vi "Send State.vi"(8 "error in (no error)":errorcluster, 11 "LV Server in":refnum<class "LV Server.lvclass">) -> (0 "error out":errorcluster, 3 "LV Server out":refnum<class "LV Server.lvclass">)   [LabVIEW 2020, in "LV Server.lvclass"]
uses:
  LV Server.lvclass
  LV Server.lvclass/LV Server.ctl
  51f6818c-cf3b-408c-aab4-b0425e769b53.vi
  Common/Message ID.ctl
  Common/Common.lvlib
  f25794c6-c553-4325-9ad1-1fe60d8e3a00.vi
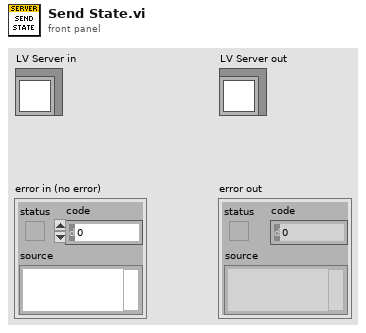
[diagram p1: front panel]
types:
  T1 = typedef "Common.lvlib/Message ID.ctl" = enum16{"Timer State", "Timer Value", "Timer Start", "Timer Pause", "Timer Reset", "Timer Init"}
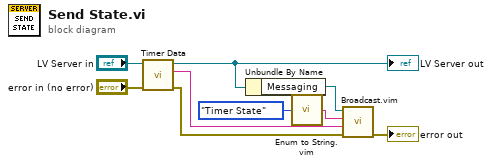
[diagram p0: block diagram]
diagram:
  n1 = call "Timer Data.vi"("error in (no error)"="error in (no error)", "LV Server in"="LV Server in") -> ("error out"=w2:errorcluster, "Timer State"=w5:string, "LV Server out"=w7:refnum<class "LV Server.lvclass">)  [unwired: 6 in, 1 out]
  "LV Server out" <- w7
  n2 = Unbundle By Name(w7) -> ("Messaging"=w6:refnum<class "Manager.lvclass">)
  n3 = call "Enum to String.vim"("Enum"=Message_ID."Timer State" ("Message ID")) -> ("Enum String"=w3:string)
  n4 = call "Broadcast.vim"("error in (no error)"=w2, "Data"=w5, "ID"=w3, "Manager in"=w6) -> ("error out"=→"error out":errorcluster)  [unwired: 6 in, 1 out]
